vi "Get VI Name.vi"(8 "error in (no error)":errorcluster, 11 "Fully Qualified VI name":string) -> (0 "error out":errorcluster, 3 "VI Name":string)   [LabVIEW 2020, in "Test Finder.lvclass"]
uses:
  Test Finder.lvclass
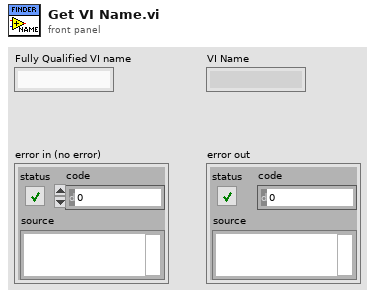
[diagram p1: front panel]
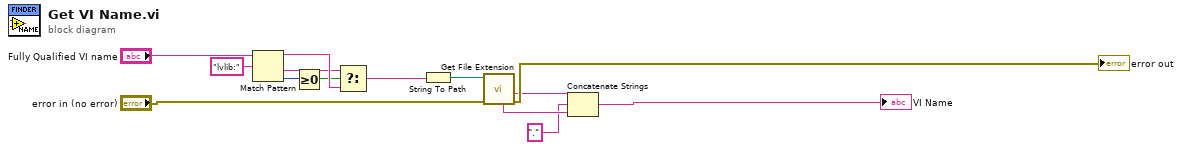
[diagram p0: block diagram]
diagram:
  n1 = Match Pattern(string="Fully Qualified VI name", regular expression="lvlib:") -> (before substring=w12:string, after substring=w11:string, offset past match=w9:i32)  [unwired: 1 in, 1 out]
  n2 = Greater Or Equal To 0?(x=w9) -> (x >= 0?=w10:bool)
  n3 = Select(t=w11, s=w10, f=w12) -> (s? t:f=w13:string)
  n4 = String To Path(string=w13) -> (path=w1:path)
  n5 = call <vilib>:"Get File Extension.vi"("error in (no error)"="error in (no error)", "file"=w1) -> ("error out"=→"error out":errorcluster, "filename without extension"=w2:string, "unmodified file extension"=w4:string)  [unwired: 5 in, 2 out]
  n6 = Concatenate Strings(w2, "." ("string"), w4) -> (→"VI Name":string)
